vi "Read.vi"(11 "GUIStateValue in":refnum<class "GUIStateValue.lvclass">) -> (2 "GUI State":T1)   [LabVIEW 2020, in "VolatusGUI.lvlib" / "GUIStateValue.lvclass"]
uses:
  GUIStateValue.lvclass
  GUI State.ctl
  <vilib>/Utility/miscctls.llb/LVRectTypeDef.ctl
  GUIStateValue.lvclass/GUIStateValue.ctl
  VolatusGUI.lvlib
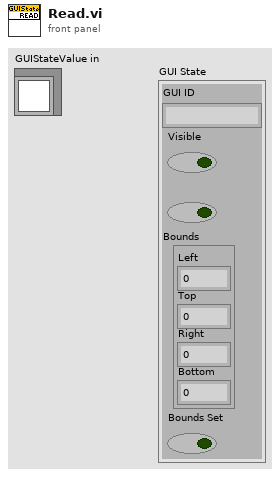
[diagram p1: front panel]
types:
  T1 = typedef "VolatusGUI.lvlib/GUI State.ctl" = cluster{"GUI ID":string, "Visible":bool, "Visibility Set":bool, "Bounds":T2, "Bounds Set":bool}
  T2 = typedef "LVRectTypeDef.ctl" = cluster{"Left":i16, "Top":i16, "Right":i16, "Bottom":i16}
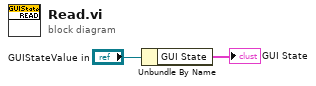
[diagram p0: block diagram]
diagram:
  n1 = Unbundle By Name("GUIStateValue in") -> ("GUI State"=→"GUI State":T1)
